vi "OpenG Filter Array vs XNode.vi"   [LabVIEW 2018]
uses:
  <userlib>/_OpenG.lib/array/array.llb/Filter 1D Array (DBL)__ogtk.vi
  <userlib>/_LAVAcr/OpenG Array XNodes/OpenG Filter Array/OpenG FilterArray.xnode
panel:
  # "This is non functional code for demonstrating the power of XNodes versus OpenG Array Nodes"
types:
  T1 = enum16{"Starwberries", "Raspberries", "Loganberries", "Tayberries", "Blackberries"}
  T2 = enum16{"Starwberries", "Raspberries", "Loganberries", "Tayberries", "Blackberries"}[]
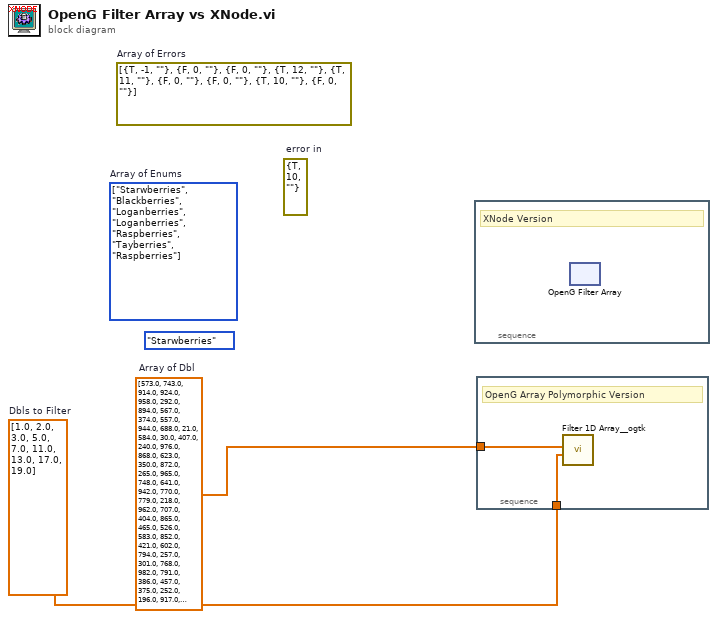
[diagram p0: block diagram]
diagram:
  (unwired) errorcluster {"status"=TRUE, "code"=10, "source"=""}  # error in
  (unwired) errorcluster[] [{"status"=TRUE, "code"=-1, "source"=""}, {"status"=FALSE, "code"=0, "source"=""}, {"status"=FALSE, "code"=0, "source"=""}, {"status"=TRUE, "code"=12, "source"=""}, {"status"=TRUE, "code"=11, "source"=""}, {"status"=FALSE, "code"=0, "source"=""}, {"status"=FALSE, "code"=0, "source"=""}, {"status"=TRUE, "code"=10, "source"=""}, {"status"=FALSE, "code"=0, "source"=""}]  # Array of Errors
  w1 = dbl[] [1.0, 2.0, 3.0, 5.0, 7.0, 11.0, 13.0, 17.0, 19.0]  # Dbls to Filter
  w2 = dbl[] [573.0, 743.0, 914.0, 924.0, 958.0, 292.0, 894.0, 567.0, 374.0, 557.0, 944.0, 688.0, 21.0, 584.0, 30.0, 407.0, 240.0, 976.0, 868.0, 623.0, 350.0, 872.0, 265.0, 965.0, 748.0, 641.0, 942.0, 770.0, 779.0, 218.0, 962.0, 707.0, 404.0, 865.0, 465.0, 526.0, 583.0, 852.0, 421.0, 602.0, 794.0, 257.0, 301.0, 768.0, 982.0, 791.0, 386.0, 457.0, 375.0, 252.0, 196.0, 917.0, 880.0, 305.0, 355.0, 3.0, 624.0, 723.0, 486.0, 132.0, 25.0, 987.0, 260.0, 975.0, 747.0, 810.0, 946.0, 258.0, 944.0, 416.0, 66.0, 440.0, 955.0, 224.0, 90.0, 811.0, 569.0, 102.0, 723.0, 839.0, 622.0, 195.0, 748.0, 59.0, 114.0, 95.0, 716.0, 617.0, 222.0, 864.0, 521.0, 737.0, 830.0, 7.0, 84.0, 388.0, 230.0, 886.0, 193.0, 336.0]  # Array of Dbl
  (unwired) T1."Starwberries" ("items to filter")
  (unwired) T2 [enum."Starwberries", enum."Blackberries", enum."Loganberries", enum."Loganberries", enum."Raspberries", enum."Tayberries", enum."Raspberries"] items=["Starwberries", "Raspberries", "Loganberries", "Tayberries", "Blackberries"]  # Array of Enums
  n1 = stacked-sequence {
    frame #0 {
      # "XNode Version"
      n2 = xnode "OpenG Filter Array"() -> ()  [unwired: 2 in, 2 out]
    }
  }
  n3 = stacked-sequence {
    tunnel: w2 -> [w4]
    tunnel: w1 -> [w3]
    frame #0 {
      # "OpenG Array Polymorphic Version"
      n4 = call-poly <userlib>:"Filter 1D Array__ogtk.vi"("items to filter"=w3, "array"=w4) -> ()  [unwired: 4 in, 2 out]
    }
  }
